vi "CRYPlot Picture Graph.vi"(10 "Flattened Property":string, 11 "pGraph VI In":refnum<vi>) -> ()   [LabVIEW 2013]
uses:
  CRYWindow/DataView/Control/CRYPicture Property.ctl
panel:
  in  "Picture Property":T1
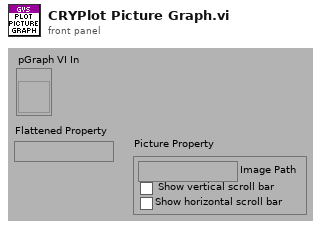
[diagram p1: front panel]
types:
  T1 = typedef "CRYPicture Property.ctl" = cluster{"Image Path":string, "Show vertical scroll bar":bool, "Show horizontal scroll bar":bool}
  T2 = typedef "imagedata.ctl" = cluster{"image type":i32, "image depth":i32, "image":u8[], "mask":u8[], "colors":u32[], "Rectangle":cluster{"left":i16, "top":i16, "right":i16, "bottom":i16}}
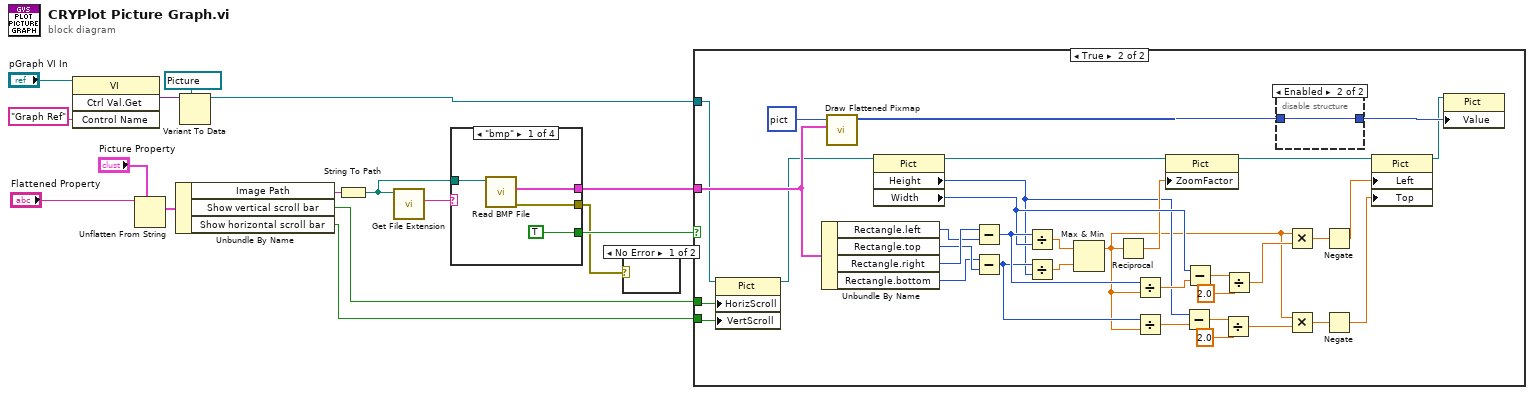
[diagram p0: block diagram]
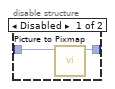
[diagram p4: hidden frame]
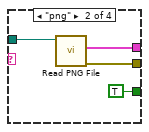
[diagram p5: hidden frame]
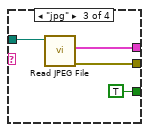
[diagram p6: hidden frame]
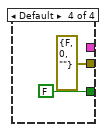
[diagram p7: hidden frame]
diagram:
  n1 = invoke class="VI" method="Ctrl Val.Get"(reference="pGraph VI In", "Control Name"="Graph Ref") -> ("Get Control Value Variant"=w2:variant)  [unwired: 2 in, 3 out]
  n2 = Unflatten From String(type="Picture Property", binary string="Flattened Property") -> (value=w10:T1)  [unwired: 3 in, 2 out]
  n3 = Unbundle By Name(w10) -> ("Image Path"=w9:string, "Show vertical scroll bar"=w8:bool, "Show horizontal scroll bar"=w7:bool)
  n4 = Variant To Data(type=refnum<vi> refnum ("Graph Ref"), Variant=w2) -> (data=w1:refnum<vi>)  [unwired: 1 in, 1 out]
  n5 = String To Path(string=w9) -> (path=w15:path)
  n6 = call <vilib>:"Get File Extension.vi"("file"=w15) -> ("lowercase file extension"=w16:string)  [unwired: 1 in, 9 out]
  n7 = case shown="\"bmp\"" w16 {
    tunnel: w15 -> [w20 w24 w28 _]
    tunnel: [w19 w23 w27 _] -> w13
    tunnel: [TRUE TRUE TRUE FALSE] -> w14
    tunnel: [w17 w21 w25 errorcluster {"status"=FALSE, "code"=0, "source"=""} ("error out")] -> w6
    frame "bmp" {
      n8 = call <vilib>:"Read BMP File.vi"("path to BMP file"=w20) -> ("error out"=w17:errorcluster, "image data"=w19:T2)  [unwired: 8 in, 1 out]
    }
    frame "png" {
      n9 = call <vilib>:"Read PNG File.vi"("path to PNG file"=w24) -> ("error out"=w21:errorcluster, "image data"=w23:T2)  [unwired: 8 in, 1 out]
    }
    frame "jpg" {
      n10 = call <vilib>:"Read JPEG File.vi"("path to JPEG file"=w28) -> ("error out"=w25:errorcluster, "image data"=w27:T2)  [unwired: 8 in, 1 out]
    }
    frame Default {
    }
  }
  n11 = case shown="No Error" w6 {
    frame No Error {
    }
    frame Error {
    }
  }
  n12 = case shown="True" w14 {
    tunnel: w13 -> [_ w56]
    tunnel: w1 -> [_ w54]
    tunnel: w8 -> [_ w53]
    tunnel: w7 -> [_ w52]
    frame False {
    }
    frame True {
      n13 = property class="Pict"(reference=w54, "HorizScroll"=w53, "VertScroll"=w52) -> (reference out=w51:refnum<vi>)  [unwired: 1 in, 1 out]
      n14 = Unbundle By Name(w56) -> ("Rectangle.left"=w59:i16, "Rectangle.top"=w58:i16, "Rectangle.right"=w60:i16, "Rectangle.bottom"=w57:i16)
      n15 = call <vilib>:"Draw Flattened Pixmap.vi"("image data"=w56, "picture"=picture data[5B]) -> ("new picture"=w64:picture)  [unwired: 7 in]
      n16 = property on="Property Node" class="Pict"(reference=w51) -> (reference out=w55:refnum<vi>, "Height"=w35:u32, "Width"=w48:u32)  [unwired: 1 in, 1 out]
      n17 = Subtract(x=w60, y=w59) -> (x-y=w50:i16)
      n18 = Subtract(x=w57, y=w58) -> (x-y=w39:i16)
      n19 = Divide(x=w50, y=w48) -> (x/y=w61:dbl)
      n20 = Divide(x=w39, y=w35) -> (x/y=w62:dbl)
      n21 = Max & Min(x=w61, y=w62) -> (max(x,y)=w32:dbl)  [unwired: 1 out]
      n22 = Reciprocal(x=w32) -> (1/x=w43:dbl)
      n23 = Divide(x=w50, y=w32) -> (x/y=w49:dbl)
      n24 = Divide(x=w39, y=w32) -> (x/y=w36:dbl)
      n25 = property class="Pict"(reference=w55, "ZoomFactor"=w43) -> (reference out=w45:refnum<vi>)  [unwired: 1 in, 1 out]
      n26 = Subtract(x=w35, y=w36) -> (x-y=w37:dbl)
      n27 = Subtract(x=w48, y=w49) -> (x-y=w47:dbl)
      n28 = Divide(x=w37, y=2.0) -> (x/y=w33:dbl)
      n29 = Divide(x=w47, y=2.0) -> (x/y=w41:dbl)
      n30 = disable-structure shown="Enabled" {
        disable-tunnel: w64 -> [w67 w68]
        disable-tunnel: [w66 w68] -> w63
        frame Disabled {
          n31 = call <vilib>:"Picture to Pixmap.vi"("picture"=w67) -> ("new picture"=w66:picture)  [unwired: 9 in, 1 out]
        }
        frame Enabled {
        }
      }
      n32 = Multiply(x=w32, y=w41) -> (x*y=w40:dbl)
      n33 = Multiply(x=w32, y=w33) -> (x*y=w34:dbl)
      n34 = Negate(x=w40) -> (-x=w42:dbl)
      n35 = Negate(x=w34) -> (-x=w31:dbl)
      n36 = property class="Pict"(reference=w45, "Left"=w42, "Top"=w31) -> (reference out=w44:refnum<vi>)  [unwired: 1 in, 1 out]
      n37 = property on="Property Node" class="Pict"(reference=w44, "Value"=w63) -> ()  [unwired: 1 in, 2 out]
    }
  }
